vi "ex2_consumer.vi"() -> ()   [LabVIEW 2022 SP3]
uses:
  pylabview/pythonq.lvlib
  C:/Program Files (x86)/National Instruments/LabVIEW 2022/examples/Connectivity/Python/support/PythonVersionsEnum.ctl
  py_msg.ctl
  pylabview/py_result.ctl
panel:
  out "response":T1
  out "v":dbl format="%.15g"
  in  "que_out?":bool=TRUE
  out "ref":string
  out "count 1":i32
  out "error out":errorcluster
  out "Wv":dbl(graph)
  in  "stop":bool
  out "count 2":i32
  # "# Created by Jeff Morgan\n# https://awakeniot.com/"
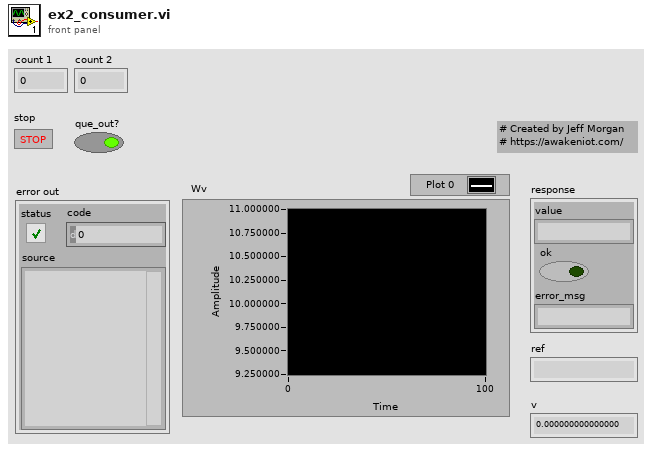
[diagram p1: front panel]
types:
  T1 = typedef "pythonq.lvlib/py_result.ctl" = cluster{"value":string, "ok":bool, "error_msg":string}
  T2 = typedef "PythonVersionsEnum.ctl" = enum16{"3.6", "3.7", "3.8", "3.9"}
  T3 = typedef "python_q.lvlib/py_cluster.ctl" = cluster{"path":path, "py":T4}
  T4 = typedef "python_q.lvlib/py_session.ctl" = cluster{"session":refnum<k35>, "object":refnum<k38>}
  T5 = typedef "pythonq.lvlib/py_cluster.ctl" = cluster{"path":path, "py":T6}
  T6 = typedef "pythonq.lvlib/py_session.ctl" = cluster{"session":refnum<k35>, "object":refnum<k38>}
  T7 = typedef "py_msg.ctl" = cluster{"double":dbl, "ref":string}
  T8 = typedef "python_q.lvlib/py_result.ctl" = cluster{"value":string, "ok":bool, "error_msg":string}
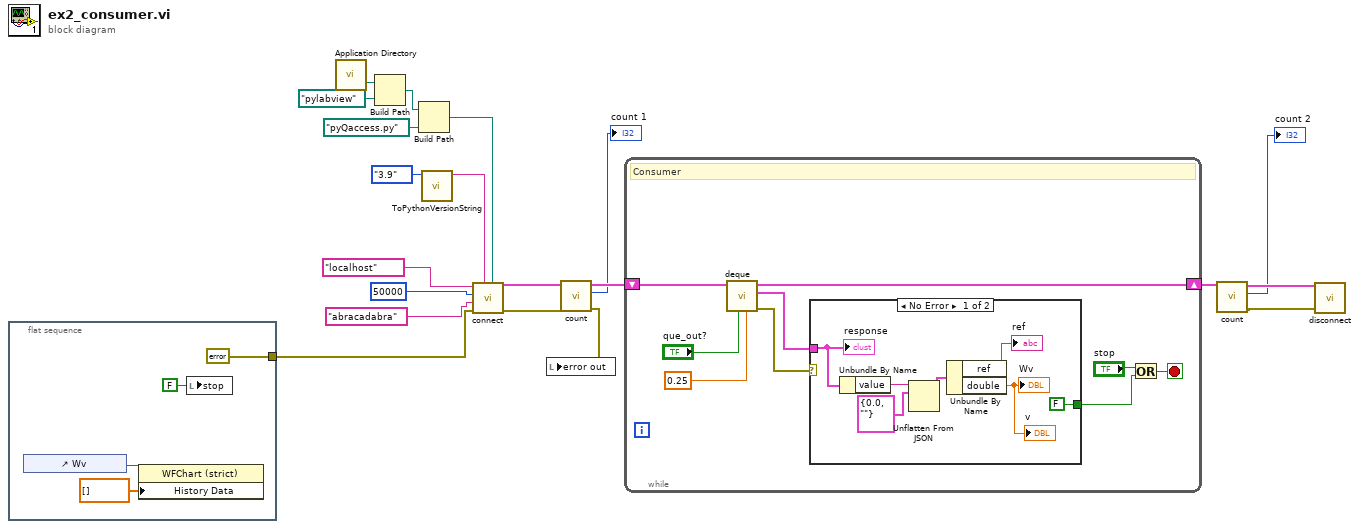
[diagram p0: block diagram]
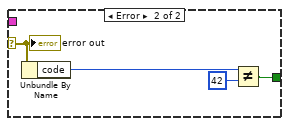
[diagram p2: hidden frame]
diagram:
  n1 = flat-sequence {
    tunnel: [errorcluster {"status"=FALSE, "code"=0, "source"=""} ("error in (no error)")] -> w3
    frame #0 {
      n2 = control-ref of="Wv"() -> (w22:refnum<vi>)
      n3 = property class="WFChart (strict)"(reference=w22, "History Data"=dbl[] []) -> ()  [unwired: 1 in, 2 out]
      n4 = local write "stop"(FALSE ("stop")) -> ()
    }
  }
  n5 = call <vilib>:"Application Directory.vi"() -> ("Application Directory"=w14:path)
  n6 = Build Path(base path=w14, name or relative path=path "pylabview") -> (appended path=w15:path)
  n7 = Build Path(base path=w15, name or relative path=path "pyQaccess.py") -> (appended path=w12:path)
  n8 = call "ToPythonVersionString.vi"("python version"=PythonVersionsEnum."3.9") -> ("python version string"=w17:string)  [unwired: 10 in]
  n9 = call "connect.vi"("module path"=w12, "Python version"=w17, "error in (no error)"=w3, "password"="abracadabra", "port"=50000, "ip_address"="localhost") -> ("error out"=w6:errorcluster, "py out"=w5:T3)  [unwired: 4 in]
  n10 = call "count.vi"("error in (no error)"=w6, "py in"=w5) -> ("error out"=w1:errorcluster, "count"=→"count 1":i32, "py out"=w4:T5)  [unwired: 7 in]
  n11 = local write "error out"(w1) -> ()
  n12 = while {
    shift-right: [w32] -> w10
    shift-left: w4 -> [w33]
    stop <- w29 stop-if-true
    # "Consumer"
    n13 = call "deque.vi"("timeout"=0.25, "que_out?"="que_out?", "py in"=w33) -> ("error out"=w30:errorcluster, "response"=w25:T8, "py out"=w32:T3)  [unwired: 5 in, 1 out]
    n14 = case shown="No Error" w30 {
      selector: w30 -> [_ w44]
      tunnel: [FALSE w41] -> w27
      tunnel: w25 -> [w39 _]
      frame No Error {
        n15 = Unbundle By Name(w39) -> ("value"=w38:string)
        n16 = Unflatten From JSON(JSON string=w38, type and defaults=T7 {"double"=0.0, "ref"=""} ("Cluster")) -> (value=w36:T7)  [unwired: 5 in, 1 out]
        n17 = Unbundle By Name(w36) -> ("ref"=→"ref":string, "double"=→"Wv" →"v":dbl)
        "response" <- w39
      }
      frame Error {
        n18 = Unbundle By Name(w44) -> ("code"=w43:i32)
        n19 = Not Equal?(x=w43, y=42) -> (x != y?=w41:bool)
        "error out" <- w44
      }
    }
    n20 = Or(x="stop", y=w27) -> (x .or. y?=w29:bool)
  }
  n21 = call "count.vi"("py in"=w10) -> ("error out"=w8:errorcluster, "count"=→"count 2":i32, "py out"=w9:T5)  [unwired: 8 in]
  n22 = call "disconnect.vi"("error in (no error)"=w8, "py in"=w9) -> ()  [unwired: 9 in, 1 out]
